vi "湿度报警.vi"(0 "选择湿度曲线":enum16{"湿度1", "湿度2", "平均湿度"}(ring)=enum."平均湿度", 1 "输出簇 2":T1, 3 "警示":refnum<vi>) -> (6 "预警":string)   [LabVIEW 2016]
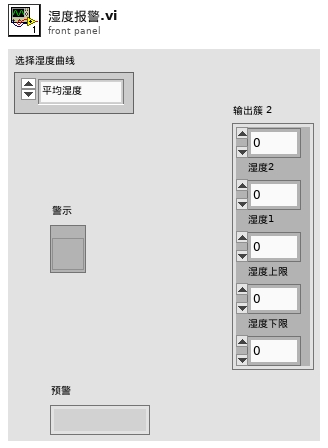
[diagram p1: front panel]
types:
  T1 = cluster{dbl, "湿度2":dbl, "湿度1":dbl, "湿度上限":dbl, "湿度下限":dbl}
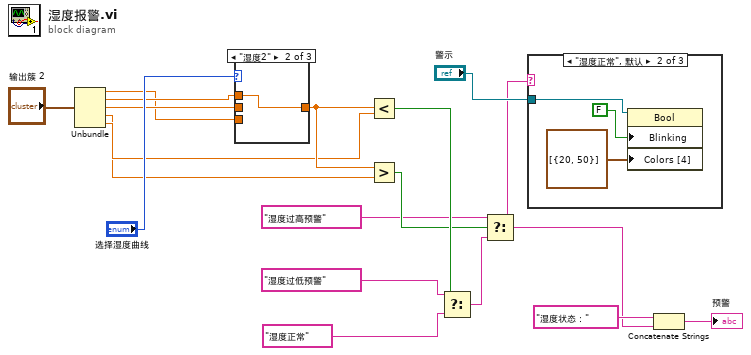
[diagram p0: block diagram]
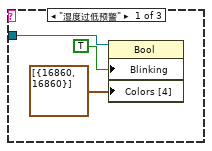
[diagram p4: hidden frame]
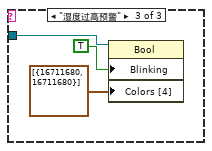
[diagram p5: hidden frame]
diagram:
  n1 = Unbundle("输出簇 2") -> (w4:dbl, "湿度2"=w5:dbl, "湿度1"=w6:dbl, "湿度上限"=w7:dbl, "湿度下限"=w8:dbl)
  n2 = case shown="\"湿度2\"" "选择湿度曲线" {
    tunnel: [w19 w20 w21] -> w10
    tunnel: w5 -> [_ w20 _]
    tunnel: w6 -> [w19 _ _]
    tunnel: w4 -> [_ _ w21]
    frame "湿度1" {
    }
    frame "湿度2" {
    }
    frame "平均湿度", Default {
    }
  }
  n3 = Less?(x=w10, y=w8) -> (x < y?=w17:bool)
  n4 = Greater?(x=w10, y=w7) -> (0:w16:bool)
  n5 = Select(t="湿度过低预警", s=w17, f="湿度正常") -> (s? t:f=w13:string)
  n6 = Select(t="湿度过高预警", s=w16, f=w13) -> (s? t:f=w2:string)
  n7 = case shown="\"湿度正常\", 默认" w2 {
    tunnel: "警示" -> [w24 w27 w30]
    frame "湿度过低预警" {
      n8 = property class="Bool"(reference=w24, "Blinking"=TRUE ("闪烁"), "Colors [4]"=cluster{u32, u32}[] [{16860, 16860}] ("颜色[4]")) -> ()  [unwired: 1 in, 2 out]
    }
    frame "湿度正常", Default {
      n9 = property class="Bool"(reference=w27, "Blinking"=FALSE ("闪烁"), "Colors [4]"=cluster{u32, u32}[] [{20, 50}] ("颜色[4]")) -> ()  [unwired: 1 in, 2 out]
    }
    frame "湿度过高预警" {
      n10 = property class="Bool"(reference=w30, "Blinking"=TRUE ("闪烁"), "Colors [4]"=cluster{u32, u32}[] [{16711680, 16711680}] ("颜色[4]")) -> ()  [unwired: 1 in, 2 out]
    }
  }
  n11 = Concatenate Strings("湿度状态：" ("字符串"), w2) -> (→"预警":string)
